vi "usb2000SetAcquireTime.vi"(8 "error in (no error)":errorcluster, 10 "Integration Time (6000)":u32=6000, 11 "VISA resource name":refnum<visa-resource-name>) -> (0 "error out":errorcluster, 2 "validIntegrationTime":i32, 3 "VISA resource name out":refnum<visa-resource-name>)   [LabVIEW 2015]
uses:
  <instrlib>/Ocean Optics 2000 4000/Ocean Optics 2000 4000.lvlib
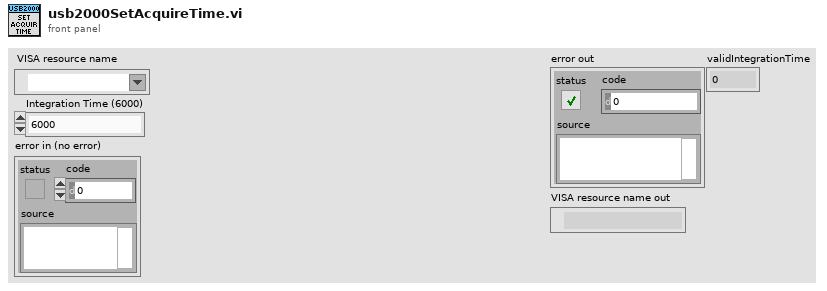
[diagram p1: front panel]
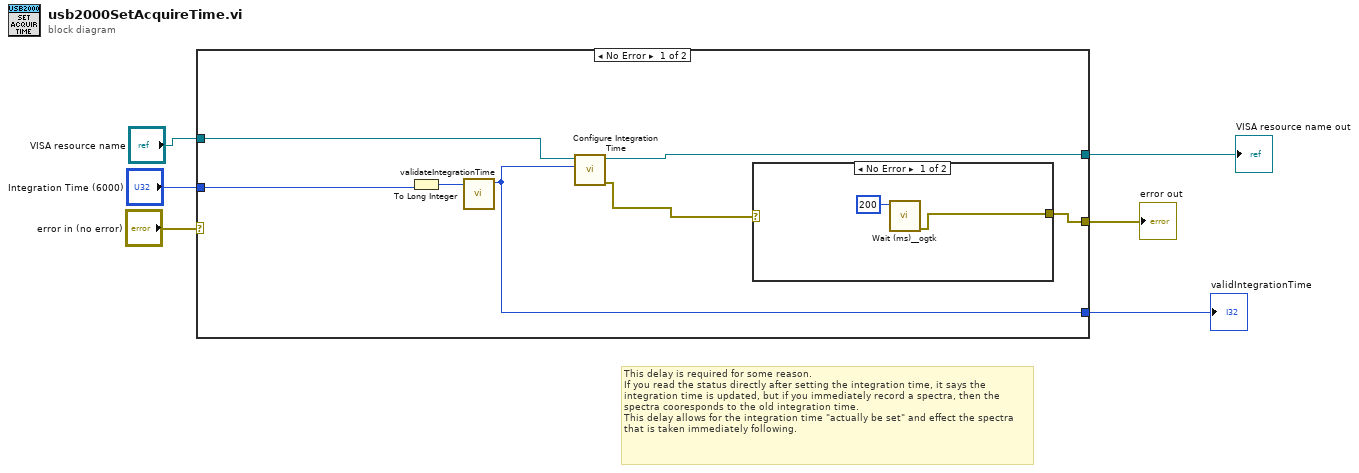
[diagram p0: block diagram]
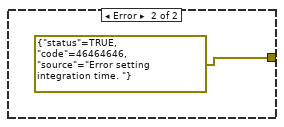
[diagram p2: hidden frame]
diagram:
  # "This delay is required for some reason. \nIf you read the status directly after setting the integration time, it says the integration time is updated, but if you immediately record a spectra, then the spectra cooresponds to the old integration time. \nThis delay allows for the integration time \"actually be set\" and effect the spectra that is taken immediately following."
  n1 = case shown="No Error" "error in (no error)" {
    selector: "error in (no error)" -> [_ w19]
    tunnel: [w9 w19] -> w5
    tunnel: "VISA resource name" -> [w13 w18]
    tunnel: [w12 w18] -> w3
    tunnel: [w8 w17] -> w2
    tunnel: "Integration Time (6000)" -> [w7 w17]
    frame No Error {
      n2 = To Long Integer(number=w7) -> (32bit integer=w11:i32)
      n3 = call "validateIntegrationTime.vi"("integrationTime"=w11) -> ("validIntegrationTime"=w8:i32)  [unwired: 10 in]
      n4 = call <instrlib>:"Configure Integration Time.vi"("Integration Time (6000)"=w8, "VISA resource name"=w13) -> ("error out"=w10:errorcluster, "VISA resource name out"=w12:refnum<visa-resource-name>)  [unwired: 1 in, 7 out]
      n5 = case shown="No Error" w10 {
        tunnel: [w14 errorcluster {"status"=TRUE, "code"=46464646, "source"="Error setting integration time. "} ("error out")] -> w9
        frame No Error {
          n6 = call <userlib>:"Wait (ms)__ogtk.vi"("milliseconds to wait"=u32 200) -> ("error out"=w14:errorcluster)  [unwired: 9 in, 1 out]
        }
        frame Error {
        }
      }
    }
    frame Error {
    }
  }
  "error out" <- w5
  "VISA resource name out" <- w3
  "validIntegrationTime" <- w2
